vi "Self Configure.vi"(8 "error in":errorcluster, 11 "FunctionGenerator in":refnum<class "FunctionGenerator.lvclass">) -> (0 "error out":errorcluster, 3 "FunctionGenerator out":refnum<class "FunctionGenerator.lvclass">)   [LabVIEW 2019, in "FunctionGenerator.lvlib" / "FunctionGenerator.lvclass"]
doc: "Children of Instruments must override this routine and call the parent method. \nThis routine is implemented to allow each instrument to read its specific configuration keys and implement any default configuration settings.\n\nThis routine already calls Connect and Self Test Routines."
uses:
  Library/FunctionGenerator.lvclass
  Custom Controls/Configuration Keys.ctl
  Library/FunctionGenerator.lvclass/FunctionGenerator.ctl
  builds/Instruments/Instruments.lvlibp/Library/Instruments.lvclass
  builds/Tools/Config.lvlibp/Config.lvclass
  C:/Users/Public/Documents/Development/builds/Tools/Config.lvlibp/Config.lvclass
panel:
  in  "Configuration Keys":T1
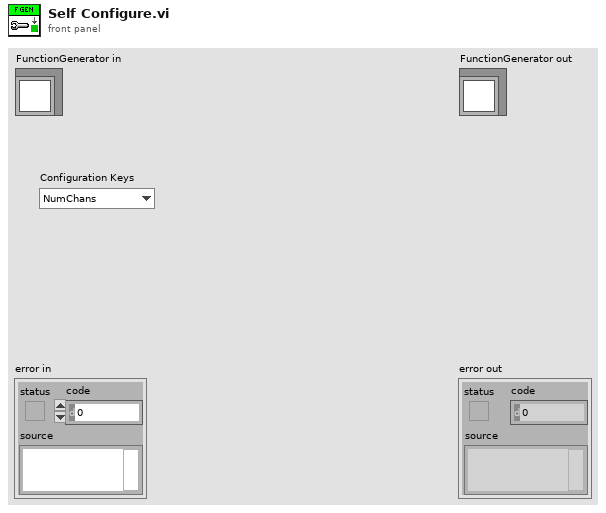
[diagram p1: front panel]
types:
  T1 = typedef "FunctionGenerator.lvlib/FunctionGenerator.lvclass/Configuration Keys.ctl" = enum16{"NumChans"}
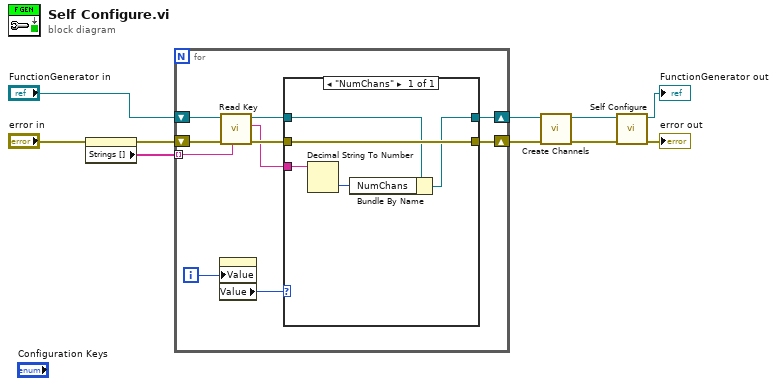
[diagram p0: block diagram]
diagram:
  n1 = property on="Configuration Keys" class="Enum (strict)"(error in="error in") -> (error out=w5:errorcluster, "Strings []"=w8:string[])  [unwired: 1 in, 1 out]
  n2 = for {
    tunnel: w8 -> [w12] mode=indexing
    shift-right: [w16] -> w4
    shift-left: "FunctionGenerator in" -> [w14]
    shift-right: [w17] -> w3
    shift-left: w5 -> [w18]
    i -> [w20]
    n3 = property on="Configuration Keys" class="Enum (strict)"("Value"=w20) -> ("Value"=w19:T1)  [unwired: 2 in, 2 out]
    n4 = call "Read Key.vi"("Key Name"=w12, "error in"=w18, "Config in"=w14) -> ("error out"=w15:errorcluster, "Key Value"=w11:string, "Config out"=w13:refnum<class "FunctionGenerator.lvclass">)  [unwired: 6 in]
    n5 = case shown="\"NumChans\"" w19 {
      tunnel: w13 -> [w24]
      tunnel: w15 -> [w25]
      tunnel: [w25] -> w17
      tunnel: [w22] -> w16
      tunnel: w11 -> [w23]
      frame "NumChans" {
        n6 = Decimal String To Number(string=w23) -> (number=w21:i32)  [unwired: 2 in, 1 out]
        n7 = Bundle By Name(cluster=w24, "NumChans"=w21) -> (w22:refnum<class "FunctionGenerator.lvclass">)
      }
    }
  }
  n8 = call "Create Channels.vi"("error in (no error)"=w3, "FunctionGenerator in"=w4) -> ("error out"=w1:errorcluster, "FunctionGenerator out"=w2:refnum<class "FunctionGenerator.lvclass">)  [unwired: 8 in]
  n9 = call-parent "Self Configure.vi"("error in"=w1, "Instruments in"=w2) -> ("error out"=→"error out":errorcluster, "Instruments out"=→"FunctionGenerator out":refnum<class "FunctionGenerator.lvclass">)  [unwired: 8 in]
